vi "liq average.vi"(11 "unsigned byte array":u8[](array[numeric])) -> (0 "Numeric 4":dbl, 1 "Numeric 3":dbl, 2 "Numeric 2":dbl, 3 "Numeric":dbl, 5 "Numeric 5":dbl)   [LabVIEW 2016]
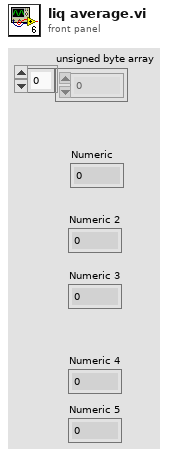
[diagram p1: front panel]
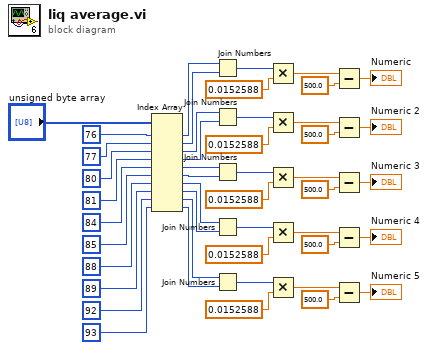
[diagram p0: block diagram]
diagram:
  n1 = Index Array(array="unsigned byte array", index #1=76 ("index"), index #2=77 ("index"), index #3=80 ("index"), index #4=81 ("index"), index #5=84 ("index"), index #6=85 ("index"), index #7=88 ("index"), index #8=89 ("index"), index #9=92 ("index"), index #10=93 ("index")) -> (element #1=w31:u8, element #2=w30:u8, element #3=w26:u8, element #4=w25:u8, element #5=w21:u8, element #6=w20:u8, element #7=w16:u8, element #8=w15:u8, element #9=w11:u8, element #10=w10:u8)
  n2 = Join Numbers(hi=w31, lo=w30) -> ((hi.lo)=w35:u16)
  n3 = Join Numbers(hi=w26, lo=w25) -> ((hi.lo)=w29:u16)
  n4 = Join Numbers(hi=w21, lo=w20) -> ((hi.lo)=w24:u16)
  n5 = Join Numbers(hi=w16, lo=w15) -> ((hi.lo)=w19:u16)
  n6 = Join Numbers(hi=w11, lo=w10) -> ((hi.lo)=w14:u16)
  n7 = Multiply(x=w35, y=0.0152588) -> (x*y=w33:dbl)
  n8 = Multiply(x=w29, y=0.0152588) -> (x*y=w27:dbl)
  n9 = Multiply(x=w24, y=0.0152588) -> (x*y=w22:dbl)
  n10 = Multiply(x=w19, y=0.0152588) -> (x*y=w17:dbl)
  n11 = Multiply(x=w14, y=0.0152588) -> (x*y=w12:dbl)
  n12 = Subtract(x=w33, y=500.0) -> (x-y=→"Numeric":dbl)
  n13 = Subtract(x=w27, y=500.0) -> (x-y=→"Numeric 2":dbl)
  n14 = Subtract(x=w22, y=500.0) -> (x-y=→"Numeric 3":dbl)
  n15 = Subtract(x=w17, y=500.0) -> (x-y=→"Numeric 4":dbl)
  n16 = Subtract(x=w12, y=500.0) -> (x-y=→"Numeric 5":dbl)
